vi "dashboard_motor_calibration.vi"() -> ()   [LabVIEW 2022 SP3]
panel:
  in  "Stop":bool
  out "Write Count":i32
  out "Read Count":i32
  in  "Reset Communication":bool
  in  "USB Port":refnum<visa-resource-name>
  out "u":dbl format="%.2g"
  out "D":dbl format="%.2g"
  out "I":dbl format="%.2g"
  out "P":dbl format="%.2g"
  in  "Tau D (s)":dbl min=0.0 max=30.0 step=0.01 format="%.2g"
  in  "Td":dbl min=0.0 max=50.0 step=0.01 format="%.2g"
  in  "Ti":dbl=100.0 min=0.0 max=100.0 step=0.01 format="%.2g"
  in  "Kc":dbl min=0.0 max=50.0 step=0.01 format="%.2g"
  out "Flag AntiWindUp":bool
  in  "Tau Encoder (s)":dbl min=0.0 max=30.0 step=0.01 format="%.2g"
  out "Error (°)":dbl
  out "Controller":cluster{" P":dbl, "I":dbl, "D":dbl, "u":dbl}(graph)
  out "Error":cluster{" error":dbl, "Filtered_error":dbl}(graph)
  in  "PWM %":dbl(slide) min=-100.0 max=100.0 step=1.0 scale=-100.0..100.0
  in  "Setpoint (RPM)":dbl(slide) min=-1500.0 max=1500.0 step=100.0 scale=-1500.0..1500.0
  in  "Manual Control":bool
  out "Enc Fase A":T1(graph)
  out "Enc Fase B":cluster{"r_sp":dbl, " r_speed":dbl}(graph)
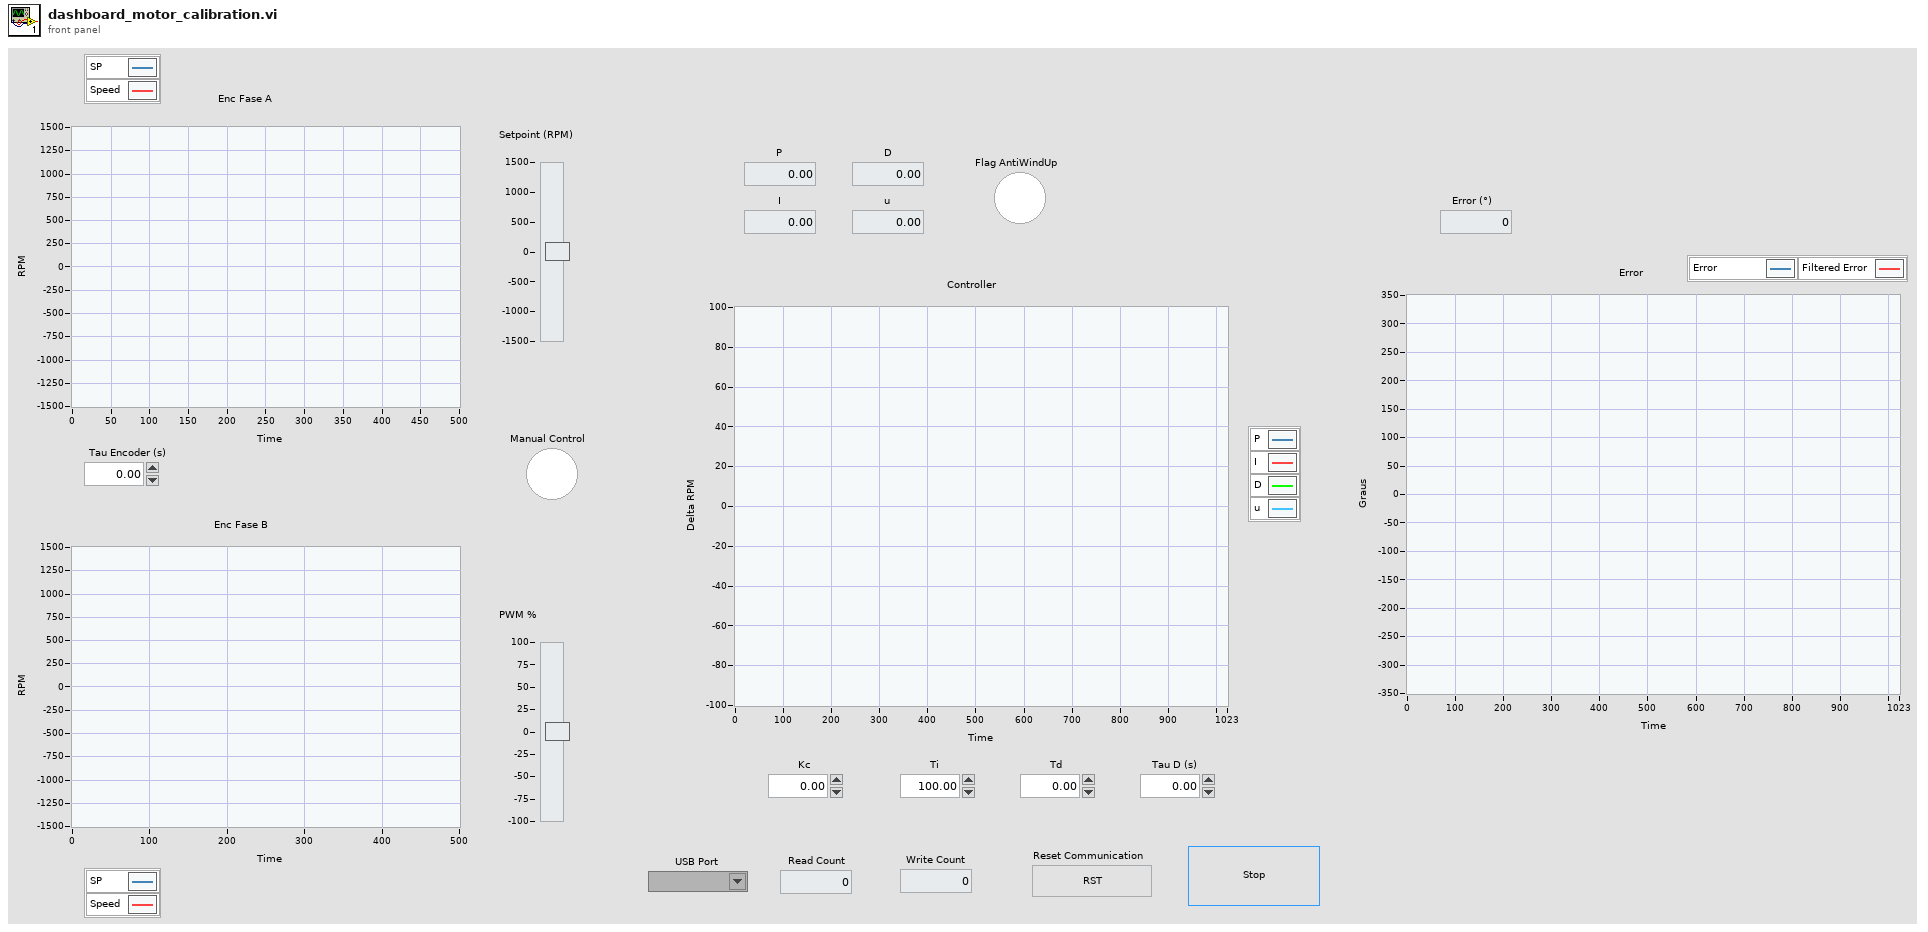
[diagram p1: front panel]
types:
  T1 = cluster{"l_sp":dbl, "l_speed":dbl, " r_speed":dbl}
  T2 = cluster{"Manual Control":bool, bool, "Setpoint (RPM)":dbl, "PWM %":dbl, "Tau Encoder (s)":dbl, "Kc":dbl, "Ti":dbl, "Td":dbl, "Tau D (s)":dbl, dbl, dbl, dbl, dbl, dbl, dbl, dbl}
  T3 = cluster{"l_sp":dbl, "l_speed":dbl, "r_sp":dbl, " r_speed":dbl, " error":dbl, "Filtered_error":dbl, " P":dbl, "I":dbl, "D":dbl, "u":dbl, "sat_flag":bool, " IR":bool[], "A_":dbl, " B_":dbl, " C_":dbl, "D_":dbl}
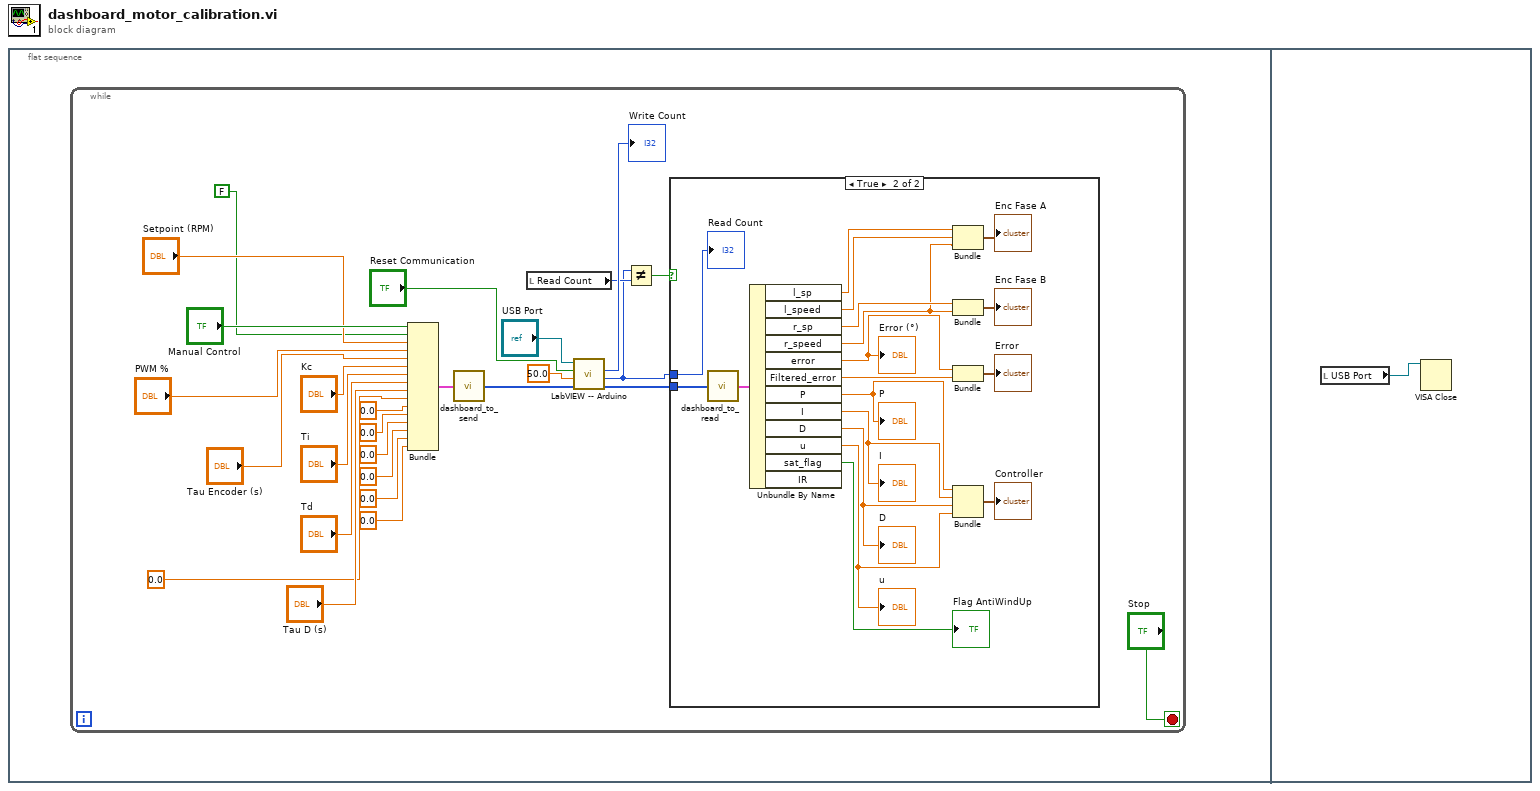
[diagram p0: block diagram]
diagram:
  n1 = flat-sequence {
    frame #0 {
      n2 = while {
        stop <- "Stop" stop-if-true
        n3 = Bundle("Manual Control"="Manual Control", FALSE, "Setpoint (RPM)"="Setpoint (RPM)", "PWM %"="PWM %", "Tau Encoder (s)"="Tau Encoder (s)", "Kc"="Kc", "Ti"="Ti", "Td"="Td", "Tau D (s)"="Tau D (s)", 0.0, 0.0, 0.0, 0.0, 0.0, 0.0, 0.0) -> (w8:T2)  [unwired: 1 in]
        n4 = call "dashboard_to_send.vi"("In"=w8) -> ("Output"=w7:u8[])
        n5 = local read "Read Count"() -> (w5:i32)
        n6 = call "LabVIEW -- Arduino.vi"("Data to Write"=w7, "Frequency Write"=50.0, "Reset"="Reset Communication", "VISA resource name"="USB Port") -> ("Read Data"=w3:u8[], "Read Count"=w4:i32, "Write Count"=→"Write Count":u16)  [unwired: 1 out]
        n7 = Not Equal?(x=w4, y=w5) -> (x != y?=w6:bool)
        n8 = case shown="True" w6 {
          tunnel: w4 -> [_ w45]
          tunnel: w3 -> [_ w44]
          frame False {
          }
          frame True {
            n9 = call "dashboard_to_read.vi"("In"=w44) -> ("Out"=w43:T3)
            n10 = Unbundle By Name(w43) -> ("l_sp"=w41:dbl, "l_speed"=w40:dbl, "r_sp"=w38:dbl, "r_speed"=w28:dbl, "error"=w34:dbl, "Filtered_error"=w33:dbl, "P"=w32:dbl, "I"=w31:dbl, "D"=w30:dbl, "u"=w29:dbl, "sat_flag"=→"Flag AntiWindUp":bool)  [unwired: 1 out]
            "Error (°)" <- w34
            "P" <- w32
            "I" <- w31
            "D" <- w30
            "u" <- w29
            n11 = Bundle("l_sp"=w41, "l_speed"=w40, "r_speed"=w28) -> (→"Enc Fase A":T1)  [unwired: 1 in]
            n12 = Bundle("r_sp"=w38, "r_speed"=w28) -> (→"Enc Fase B":cluster{"r_sp":dbl, " r_speed":dbl})  [unwired: 1 in]
            n13 = Bundle("error"=w34, "Filtered_error"=w33) -> (→"Error":cluster{" error":dbl, "Filtered_error":dbl})  [unwired: 1 in]
            n14 = Bundle("P"=w32, "I"=w31, "D"=w30, "u"=w29) -> (→"Controller":cluster{" P":dbl, "I":dbl, "D":dbl, "u":dbl})  [unwired: 1 in]
            "Read Count" <- w45
          }
        }
      }
    }
    frame #1 {
      n15 = local read "USB Port"() -> (w46:refnum<visa-resource-name>)
      n16 = VISA Close(VISA resource name=w46) -> ()  [unwired: 1 in, 1 out]
    }
  }
